vi "Lvi Set Trigger.vi"(7 "AnalogThreshold":dbl, 8 "error in (no error)":errorcluster, 9 "Polarity":u32, 10 "TrigType":u32, 11 "TaskRef":i32) -> (0 "error out":errorcluster, 2 "function return":u32(ring), 3 "TaskRef out":i32)   [LabVIEW 2022 SP3, in "DtLvLink.lvlib"]
doc: "Calls directly into the entry points of the DLL of the Data Acq SDK to specify the trigger-related attributes for an analog input or analog output task. This VI is used by the higher-level VIs, DtOLTrigger and DtOLTriggerSource."
uses:
  DtLvLink.lvlib
  <userlib>/LV-Link3/DtLvLink_64.dll
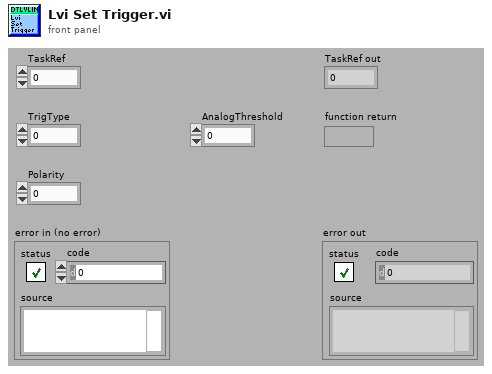
[diagram p1: front panel]
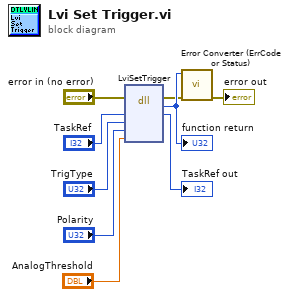
[diagram p0: block diagram]
diagram:
  n1 = dll-call lib="C:/Program Files/National Instruments/LabVIEW 2022/user.lib/LV-Link3/DtLvLink_64.*" fn="LviSetTrigger"(error in="error in (no error)", "TaskRef"="TaskRef", "TrigType"="TrigType", "Polarity"="Polarity", "AnalogThreshold"="AnalogThreshold") -> (error out=w2:errorcluster, w9:u32, "TaskRef"=→"TaskRef out":i32)  [unwired: 5 in, 1 out]
  "function return" <- w9
  n2 = call "Error Converter (ErrCode or Status).vi"("error in (no error)"=w2, "error code"=w9) -> ("error out"=→"error out":errorcluster)  [unwired: 9 in]
